vi "Com Port Request.vi"(8 "error in":errorcluster, 10 "Command":string, 11 "Com Port In":refnum<visa-resource-name>) -> (0 "error out":errorcluster, 2 "Respond":string, 3 "Com Port Out":refnum<visa-resource-name>)   [LabVIEW 2018]
uses:
  <userlib>/_MGI/Timing/MGI Wait/MGI Wait (U32).vi
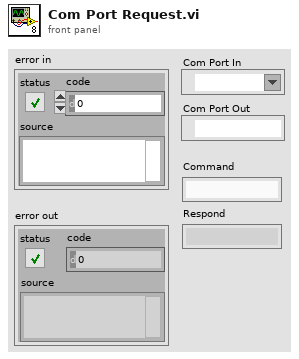
[diagram p1: front panel]
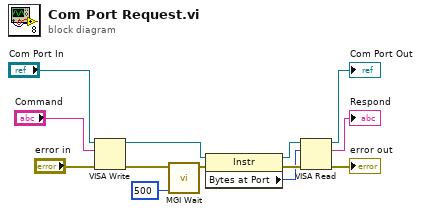
[diagram p0: block diagram]
diagram:
  n1 = VISA Write(VISA resource name="Com Port In", write buffer="Command", error in (no error)="error in") -> (VISA resource name out=w10:refnum<visa-resource-name>, error out=w13:errorcluster)  [unwired: 1 out]
  n2 = call-poly <userlib>:"MGI Wait.vi"("ms"=u32 500, "Error In"=w13) -> ("Error Out"=w11:errorcluster)  [unwired: 5 in]
  n3 = property class="Instr"(reference=w10, error in=w11) -> (reference out=w8:refnum<visa-resource-name>, error out=w9:errorcluster, "Bytes at Port"=w7:u32)
  n4 = VISA Read(VISA resource name=w8, byte count=w7, error in (no error)=w9) -> (VISA resource name out=→"Com Port Out":refnum<visa-resource-name>, read buffer=→"Respond":string, error out=→"error out":errorcluster)  [unwired: 1 out]
